vi "AttrMap-GetValue-CORE-String.vi"(8 "error in (no error)":errorcluster, 10 "Key":string, 11 "AttrMap in":T1) -> (0 "error out":errorcluster, 1 "found":bool, 2 "Value":string, 3 "AttrMap out":T1, 4 "OrgKey String":string)   [LabVIEW 2019, in "lv-apt-json-file.lvlib"]
uses:
  lv-apt-json-file.lvlib
  Typedef/Def-AttrMap.ctl
  <vilib>/addons/_JKI.lib/Serialization/JSON/JKI JSON Serialization.lvlib
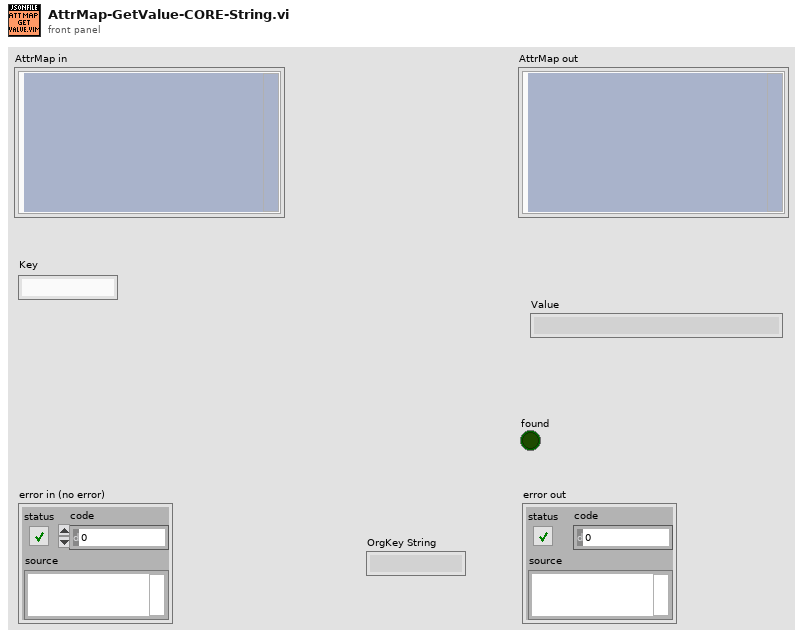
[diagram p1: front panel]
types:
  T1 = typedef "lv-apt-json-file.lvlib/Def-AttrMap.ctl" = cluster{"Map":variant}
  T2 = typedef "lv-apt-json-file.lvlib/Def-AttrMap -- NameMap.ctl" = map{string, string}
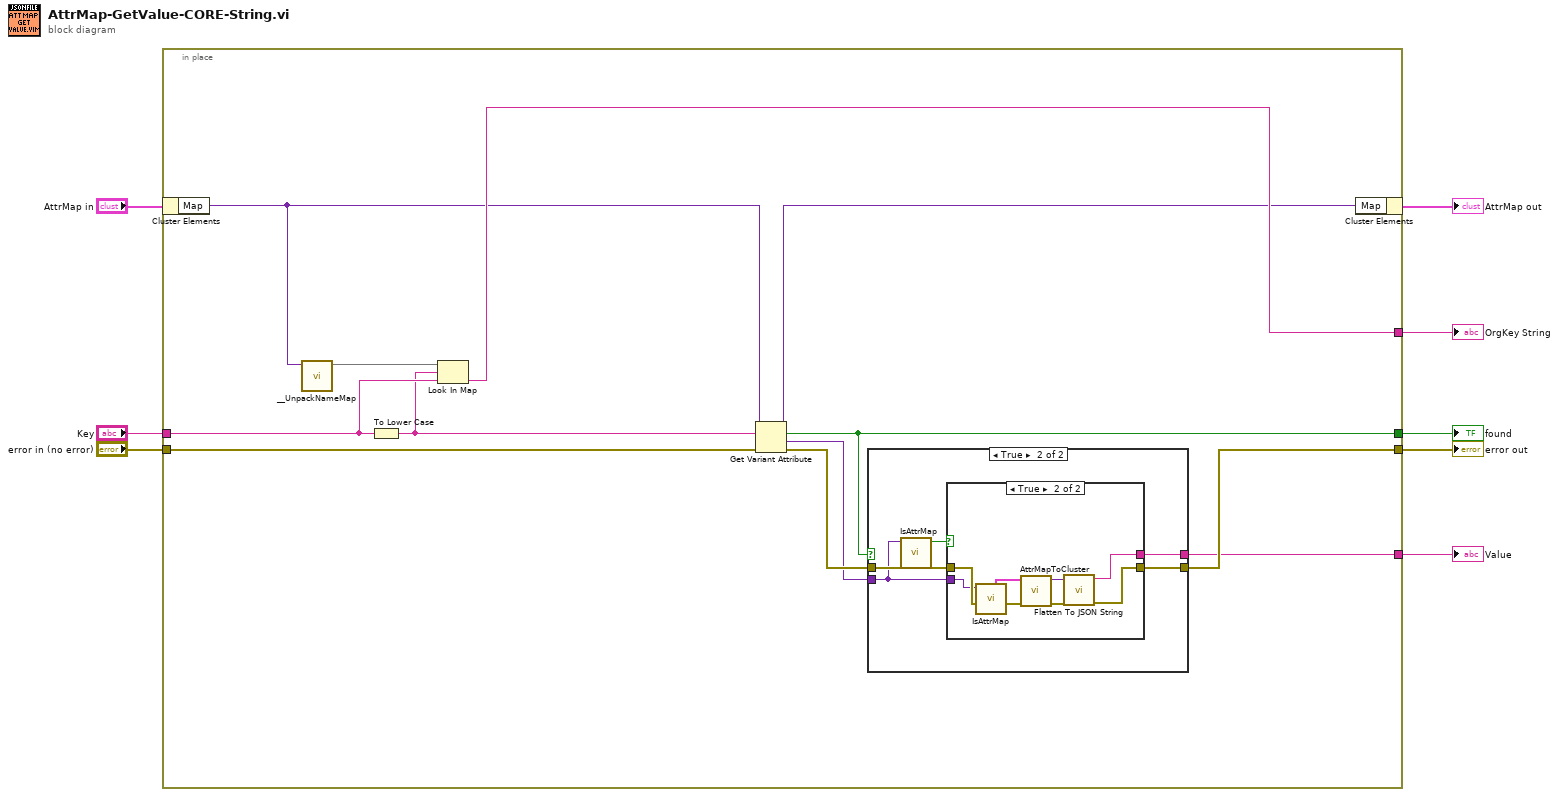
[diagram p0: block diagram]
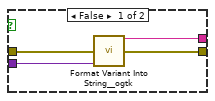
[diagram p3: hidden frame]
diagram:
  n1 = in-place {
    in-place-border: [w20] -> w8
    in-place-border: [w19] -> w7
    in-place-border: [w18] -> w6
    in-place-border: "Key" -> [w17]
    in-place-border: "error in (no error)" -> [w16]
    in-place-border: [w15] -> w3
    n2 = in-place-cluster #1("AttrMap in") -> ("Map"=w12:variant)
    n3 = call "__UnpackNameMap.vi"("Map"=w12) -> ("NameMap"=w13:T2)  [unwired: 10 in]
    n4 = To Lower Case(string=w17) -> (all lower case string=w11:string)
    n5 = Look In Map(map=w13, key=w11, default value=w17) -> (value=w15:string)  [unwired: 1 out]
    n6 = Get Variant Attribute(Variant=w12, name=w11, error in=w16) -> (duplicate Variant=w14:variant, found=w18:bool, value=w9:variant, error out=w10:errorcluster)  [unwired: 1 in]
    n7 = case shown="True" w18 {
      tunnel: [_ w26] -> w19
      tunnel: w10 -> [w21 w25]
      tunnel: [w21 w24] -> w20
      tunnel: w9 -> [_ w22]
      frame False {
      }
      frame True {
        n8 = call "IsAttrMap.vi"("Variant"=w22) -> ("True"=w23:bool)  [unwired: 8 in, 2 out]
        n9 = case shown="True" w23 {
          tunnel: [w30 w34] -> w26
          tunnel: w25 -> [w29 w37]
          tunnel: [w28 w33] -> w24
          tunnel: w22 -> [w27 w32]
          frame False {
            n10 = call <userlib>:"Format Variant Into String__ogtk.vi"("error in (no error)"=w29, "Variant"=w27) -> ("Output String"=w30:string, "error out"=w28:errorcluster)  [unwired: 12 in]
          }
          frame True {
            n11 = call "IsAttrMap.vi"("Variant"=w32) -> ("AttrMap"=w31:T1)  [unwired: 8 in, 2 out]
            n12 = call "AttrMapToCluster.vi"("error in (no error)"=w37, "AttrMap"=w31) -> ("error out"=w36:errorcluster, "Cluster"=w35:variant)  [unwired: 8 in]
            n13 = call <vilib>:"Flatten To JSON String.vi"("error in (no error)"=w36, "Variant"=w35) -> ("error out"=w33:errorcluster, "JSON String"=w34:string)  [unwired: 8 in]
          }
        }
      }
    }
    n14 = in-place-cluster #1("Map"=w14) -> (→"AttrMap out":T1)
  }
  "error out" <- w8
  "Value" <- w7
  "found" <- w6
  "OrgKey String" <- w3
